vi "config_curve.vi"(10 "簇":T23, 11 "配置":T1 {"串口通信UI"."Format" items=["标准帧", "扩展帧"]; "串口通信UI"."Type" items=["数据帧", "远程帧"]; "串口通信UI"."ID" format="0x%x"; "串口通信UI"."Fliter" items=["接收所有类型"=1, "只接收标准帧"=2, "只接收扩展帧"=3]; "串口通信UI"."kBaudRate" items=["5k bps"=1, "10k bps"=2, "20k bps"=3, "40k bps"=4, "50k bps"=5, "80k bps"=6, "100k bps"=7, "125k bps"=8, "200k bps"=9, "250k bps"=10, "400k bps"=11, "500k bps"=12, "666k bps"=13, "800k bps"=14, "1000k bps"=15, "33.33k bps"=16, "66.66k bps"=17, "83.33k bps"=18]; "串口通信UI"."Mode" items=["正常工作", "仅侦听模式", "自测模式（环回）"]; "串口通信UI"."InitFlag" items=["使用界面设置参数"=1]; "串口通信UI"."AccMask" format="%08x"; "串口通信UI"."AccCode" format="%08x"; "串口通信UI"."Channel" items=["通道1", "通道2"]; "串口通信UI"."DevType" items=["USB-CAN"=3, "USB-CAN2"=4]; "安全报警UI"."操作 8" items=["产生报警信息（不发声），等待手动操作", "产生报警信息（发声），等待手动操作", "产生报警信息（不发声），自动刹车", "产生报警信息（发声），自动刹车", "产生报警信息（不发声），立即自动断电，开启泄放电阻", "产生报警信息（发声），立即自动断电，开启泄放电阻"]; "安全报警UI"."操作 7" items=["产生报警信息（不发声），等待手动操作", "产生报警信息（发声），等待手动操作", "产生报警信息（不发声），自动刹车", "产生报警信息（发声），自动刹车", "产生报警信息（不发声），立即自动断电，开启泄放电阻", "产生报警信息（发声），立即自动断电，开启泄放电阻"]; "安全报警UI"."操作 6" items=["产生报警信息（不发声），等待手动操作", "产生报警信息（发声），等待手动操作", "产生报警信息（不发声），自动刹车", "产生报警信息（发声），自动刹车", "产生报警信息（不发声），立即自动断电，开启泄放电阻", "产生报警信息（发声），立即自动断电，开启泄放电阻"]; "安全报警UI"."操作 5" items=["产生报警信息（不发声），等待手动操作", "产生报警信息（发声），等待手动操作", "产生报警信息（不发声），自动刹车", "产生报警信息（发声），自动刹车", "产生报警信息（不发声），立即自动断电，开启泄放电阻", "产生报警信息（发声），立即自动断电，开启泄放电阻"]; "安全报警UI"."操作 4" items=["产生报警信息（不发声），等待手动操作", "产生报警信息（发声），等待手动操作", "产生报警信息（不发声），自动刹车", "产生报警信息（发声），自动刹车", "产生报警信息（不发声），立即自动断电，开启泄放电阻", "产生报警信息（发声），立即自动断电，开启泄放电阻"]; "安全报警UI"."操作 3" items=["产生报警信息（不发声），等待手动操作", "产生报警信息（发声），等待手动操作", "产生报警信息（不发声），自动刹车", "产生报警信息（发声），自动刹车", "产生报警信息（不发声），立即自动断电，开启泄放电阻", "产生报警信息（发声），立即自动断电，开启泄放电阻"]; "安全报警UI"."操作 2" items=["产生报警信息（不发声），等待手动操作", "产生报警信息（发声），等待手动操作", "产生报警信息（不发声），自动刹车", "产生报警信息（发声），自动刹车", "产生报警信息（不发声），立即自动断电，开启泄放电阻", "产生报警信息（发声），立即自动断电，开启泄放电阻"]; "安全报警UI"."操作" items=["产生报警信息（不发声），等待手动操作", "产生报警信息（发声），等待手动操作", "产生报警信息（不发声），自动刹车", "产生报警信息（发声），自动刹车", "产生报警信息（不发声），立即自动断电，开启泄放电阻", "产生报警信息（发声），立即自动断电，开启泄放电阻"]}) -> (3 "配置输出":T1 {"串口通信UI"."Format" items=["标准帧", "扩展帧"]; "串口通信UI"."Type" items=["数据帧", "远程帧"]; "串口通信UI"."ID" format="0x%x"; "串口通信UI"."Fliter" items=["接收所有类型"=1, "只接收标准帧"=2, "只接收扩展帧"=3]; "串口通信UI"."kBaudRate" items=["5k bps"=1, "10k bps"=2, "20k bps"=3, "40k bps"=4, "50k bps"=5, "80k bps"=6, "100k bps"=7, "125k bps"=8, "200k bps"=9, "250k bps"=10, "400k bps"=11, "500k bps"=12, "666k bps"=13, "800k bps"=14, "1000k bps"=15, "33.33k bps"=16, "66.66k bps"=17, "83.33k bps"=18]; "串口通信UI"."Mode" items=["正常工作", "仅侦听模式", "自测模式（环回）"]; "串口通信UI"."InitFlag" items=["使用界面设置参数"=1]; "串口通信UI"."AccMask" format="%08x"; "串口通信UI"."AccCode" format="%08x"; "串口通信UI"."Channel" items=["通道1", "通道2"]; "串口通信UI"."DevType" items=["USB-CAN"=3, "USB-CAN2"=4]; "安全报警UI"."操作 8" items=["产生报警信息（不发声），等待手动操作", "产生报警信息（发声），等待手动操作", "产生报警信息（不发声），自动刹车", "产生报警信息（发声），自动刹车", "产生报警信息（不发声），立即自动断电，开启泄放电阻", "产生报警信息（发声），立即自动断电，开启泄放电阻"]; "安全报警UI"."操作 7" items=["产生报警信息（不发声），等待手动操作", "产生报警信息（发声），等待手动操作", "产生报警信息（不发声），自动刹车", "产生报警信息（发声），自动刹车", "产生报警信息（不发声），立即自动断电，开启泄放电阻", "产生报警信息（发声），立即自动断电，开启泄放电阻"]; "安全报警UI"."操作 6" items=["产生报警信息（不发声），等待手动操作", "产生报警信息（发声），等待手动操作", "产生报警信息（不发声），自动刹车", "产生报警信息（发声），自动刹车", "产生报警信息（不发声），立即自动断电，开启泄放电阻", "产生报警信息（发声），立即自动断电，开启泄放电阻"]; "安全报警UI"."操作 5" items=["产生报警信息（不发声），等待手动操作", "产生报警信息（发声），等待手动操作", "产生报警信息（不发声），自动刹车", "产生报警信息（发声），自动刹车", "产生报警信息（不发声），立即自动断电，开启泄放电阻", "产生报警信息（发声），立即自动断电，开启泄放电阻"]; "安全报警UI"."操作 4" items=["产生报警信息（不发声），等待手动操作", "产生报警信息（发声），等待手动操作", "产生报警信息（不发声），自动刹车", "产生报警信息（发声），自动刹车", "产生报警信息（不发声），立即自动断电，开启泄放电阻", "产生报警信息（发声），立即自动断电，开启泄放电阻"]; "安全报警UI"."操作 3" items=["产生报警信息（不发声），等待手动操作", "产生报警信息（发声），等待手动操作", "产生报警信息（不发声），自动刹车", "产生报警信息（发声），自动刹车", "产生报警信息（不发声），立即自动断电，开启泄放电阻", "产生报警信息（发声），立即自动断电，开启泄放电阻"]; "安全报警UI"."操作 2" items=["产生报警信息（不发声），等待手动操作", "产生报警信息（发声），等待手动操作", "产生报警信息（不发声），自动刹车", "产生报警信息（发声），自动刹车", "产生报警信息（不发声），立即自动断电，开启泄放电阻", "产生报警信息（发声），立即自动断电，开启泄放电阻"]; "安全报警UI"."操作" items=["产生报警信息（不发声），等待手动操作", "产生报警信息（发声），等待手动操作", "产生报警信息（不发声），自动刹车", "产生报警信息（发声），自动刹车", "产生报警信息（不发声），立即自动断电，开启泄放电阻", "产生报警信息（发声），立即自动断电，开启泄放电阻"]})   [LabVIEW 2018, in "UI.lvlib"]
uses:
  UI.lvlib
  Logging/Logging Configuration.ctl
  Logging/Logging.lvlib
  Acquisition/Signal Type.ctl
  Acquisition/Acquisition.lvlib
  Acquisition/Hardware Configuration.ctl
  Settings/Settings.ctl
  Settings/Settings.lvlib
panel:
  # "参数配置文件"
  # "输入数据文件"
  # "加载电机"
  # "负载电机"
  # "注：每次运行实验时销毁现有所有图像"
  # "参数配置文件"
  # "输入数据文件"
  # "加载电机"
  # "负载电机"
  # "注：每次运行实验时销毁现有所有图像"
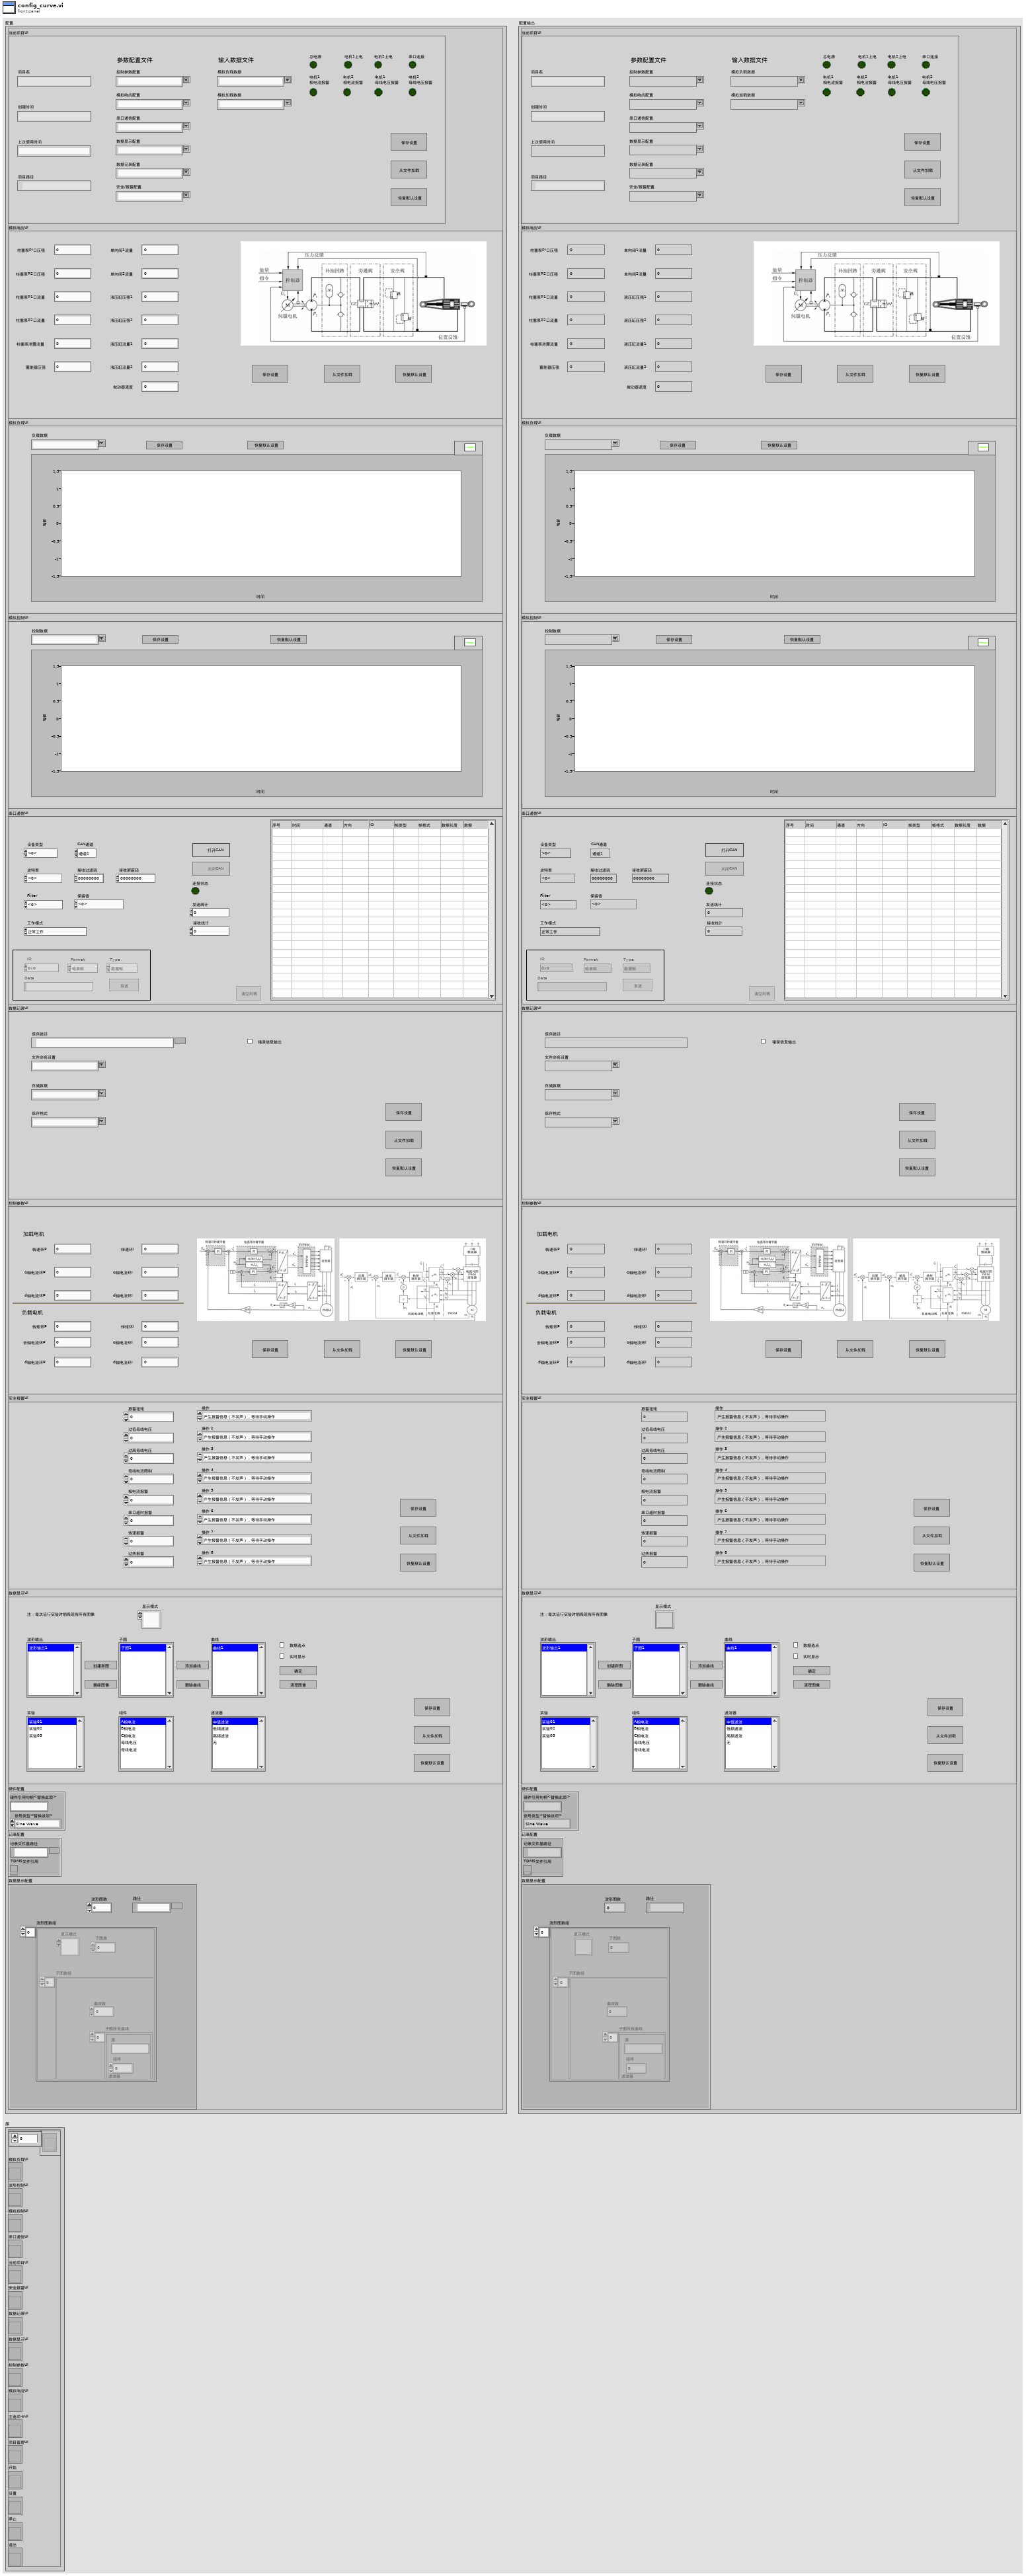
[diagram p1: front panel]
types:
  T1 = typedef "Settings.lvlib/Settings.ctl" = cluster{"当前项目UI":T2, "模拟响应UI":T3, "模拟负载UI":T4, "模拟控制UI":T5, "串口通信UI":T6, "数据记录UI":T12, "控制参数UI":T13, "安全报警UI":T14, "数据显示UI":T15, "硬件配置":T16, "记录配置":T18, "数据显示配置":T19}
  T2 = typedef "控件 5.ctl" = cluster{"控制参数配置":string, "模拟响应配置":string, "串口通信配置":string, "数据显示配置":string, "数据记录配置":string, "安全/报警配置":string, "模拟负载数据":string, "模拟加载数据":string, "总电源":bool, "电机1上电":bool, "电机2上电":bool, "串口连接":bool, "电机1\n相电流报警":bool, "电机2\n相电流报警":bool, "电机1\n母线电压报警":bool, "电机2\n母线电压报警":bool, "保存设置":bool, "从文件加载":bool, "恢复默认设置":bool, "路径":path, "项目路径":path, "项目名":string, "创建时间":string, "上次使用时间":string}
  T3 = typedef "模拟响应UI.ctl" = cluster{"柱塞泵P!口压强":dbl, "柱塞泵P2口压强":dbl, "柱塞泵P1口流量":dbl, "柱塞泵P2口流量":dbl, "柱塞泵泄露流量":dbl, "蓄能器压强":dbl, "单向阀1流量":dbl, "单向阀2流量":dbl, "液压缸压强1":dbl, "液压缸压强2":dbl, "液压缸流量1":dbl, "液压缸流量2":dbl, "做动器速度":dbl, "保存设置":bool, "从文件加载":bool, "恢复默认设置":bool, "路径":path}
  T4 = typedef "控件 9.ctl" = cluster{"负载数据":string, "负载数据 2":waveform(dbl)[], "保存设置":bool, "恢复默认设置":bool}
  T5 = typedef "控件 7.ctl" = cluster{"控制数据":string, "负载数据 2":waveform(dbl)[], "保存设置":bool, "恢复默认设置":bool}
  T6 = typedef "控件 6.ctl" = cluster{"DevType":T7, "Channel":T8, "AccCode":u32, "AccMask":u32, "InitFlag":T9, "Mode":T10, "kBaudRate":u8, "Fliter":T11, "Open":bool, "Close":bool, "连接状态":bool, "SendCnt":u32, "RecvCnt":u32, "Send":bool, "ID":u32, "Data":string, "Type":u8, "Format":u8, "Clear":bool, "list":i32, "路径":path}
  T7 = typedef "ControlCAN.lvlib/DevType.ctl" = u32
  T8 = typedef "ControlCAN.lvlib/CAN Channel.ctl" = u32
  T9 = typedef "ControlCAN.lvlib/InitFlag.ctl" = u32
  T10 = typedef "ControlCAN.lvlib/Mode.ctl" = u8
  T11 = typedef "ControlCAN.lvlib/Fliter.ctl" = u8
  T12 = typedef "控件 3.ctl" = cluster{"保存路径":path, "文件命名设置":string, "存储数据":string, "保存格式":string, "复选框":bool, "保存设置":bool, "从文件加载":bool, "恢复默认设置":bool, "路径":path}
  T13 = typedef "控件 1.ctl" = cluster{"d轴电流环P":dbl, "转速环P":dbl, "q轴电流环P":dbl, "d轴电流环P":dbl, "转矩环P":dbl, "去轴电流环P":dbl, "转速环I":dbl, "q轴电流环I":dbl, "d轴电流环I":dbl, "转矩环I":dbl, "q轴电流环I":dbl, "d轴电流环I":dbl, "保存设置":bool, "从文件加载":bool, "恢复默认设置":bool, "路径":path}
  T14 = typedef "控件 4.ctl" = cluster{"报警扭矩":dbl, "过低母线电压":dbl, "过高母线电压":dbl, "母线电流限制":dbl, "相电流报警":dbl, "串口超时报警":dbl, "转速报警":dbl, "过热报警":dbl, "操作":u16, "操作 2":u16, "操作 3":u16, "操作 4":u16, "操作 5":u16, "操作 6":u16, "操作 7":u16, "操作 8":u16, "保存设置":bool, "从文件加载":bool, "恢复默认设置":bool, "路径":path}
  T15 = typedef "控件 2.ctl" = cluster{"保存设置":bool, "从文件加载":bool, "恢复默认设置":bool, "实验":i32, "波形输出":i32, "组件":i32, "曲线":i32, "滤波器":i32, "删除曲线":bool, "清理图像":bool, "添加曲线":bool, "数据选点":bool, "确定按钮":bool, "实时显示":bool, "子图":i32, "显示模式":u16, "路径":path, "删除图像":bool, "创建新图":bool}
  T16 = typedef "Acquisition.lvlib/Hardware Configuration.ctl" = cluster{"硬件引用句柄<替换此项>":string, "信号类型<替换该项>":T17}
  T17 = typedef "Acquisition.lvlib/Signal Type.ctl" = enum16{"Sine Wave", "Square with Noise"}
  T18 = typedef "Logging.lvlib/Logging Configuration.ctl" = cluster{"记录文件基路径":path, "TDMS文件引用":refnum<k34>}
  T19 = typedef "波形图簇.ctl" = cluster{"波形图数":u32, "波形图数组":T20[], "路径":path}
  T20 = typedef "波形图.ctl" = cluster{"显示模式":u16, "子图数":u32, "子图数组":T21[]}
  T21 = typedef "子图.ctl" = cluster{"子图所有曲线":T22[], "曲线数":u32}
  T22 = typedef "曲线簇.ctl" = cluster{"源":string, "组件":u32, "滤波器":string}
  T23 = typedef "引用簇.ctl" = cluster{"数组":refnum<vi>[], "模拟负载UI":refnum<vi>, "波形控制UI":refnum<vi>, "模拟控制UI":refnum<vi>, "串口通信UI":refnum<vi>, "当前项目UI":refnum<vi>, "安全报警UI":refnum<vi>, "数据记录UI":refnum<vi>, "数据显示UI":refnum<vi>, "控制参数UI":refnum<vi>, "模拟响应UI":refnum<vi>, "主选项卡UI":refnum<vi>, "项目管理UI":refnum<vi>, "开始":refnum<vi>, "设置":refnum<vi>, "停止":refnum<vi>, "退出":refnum<vi>}
  T24 = typedef "组件常量.ctl" = string[]
  T25 = typedef "滤波器常量.ctl" = string[]
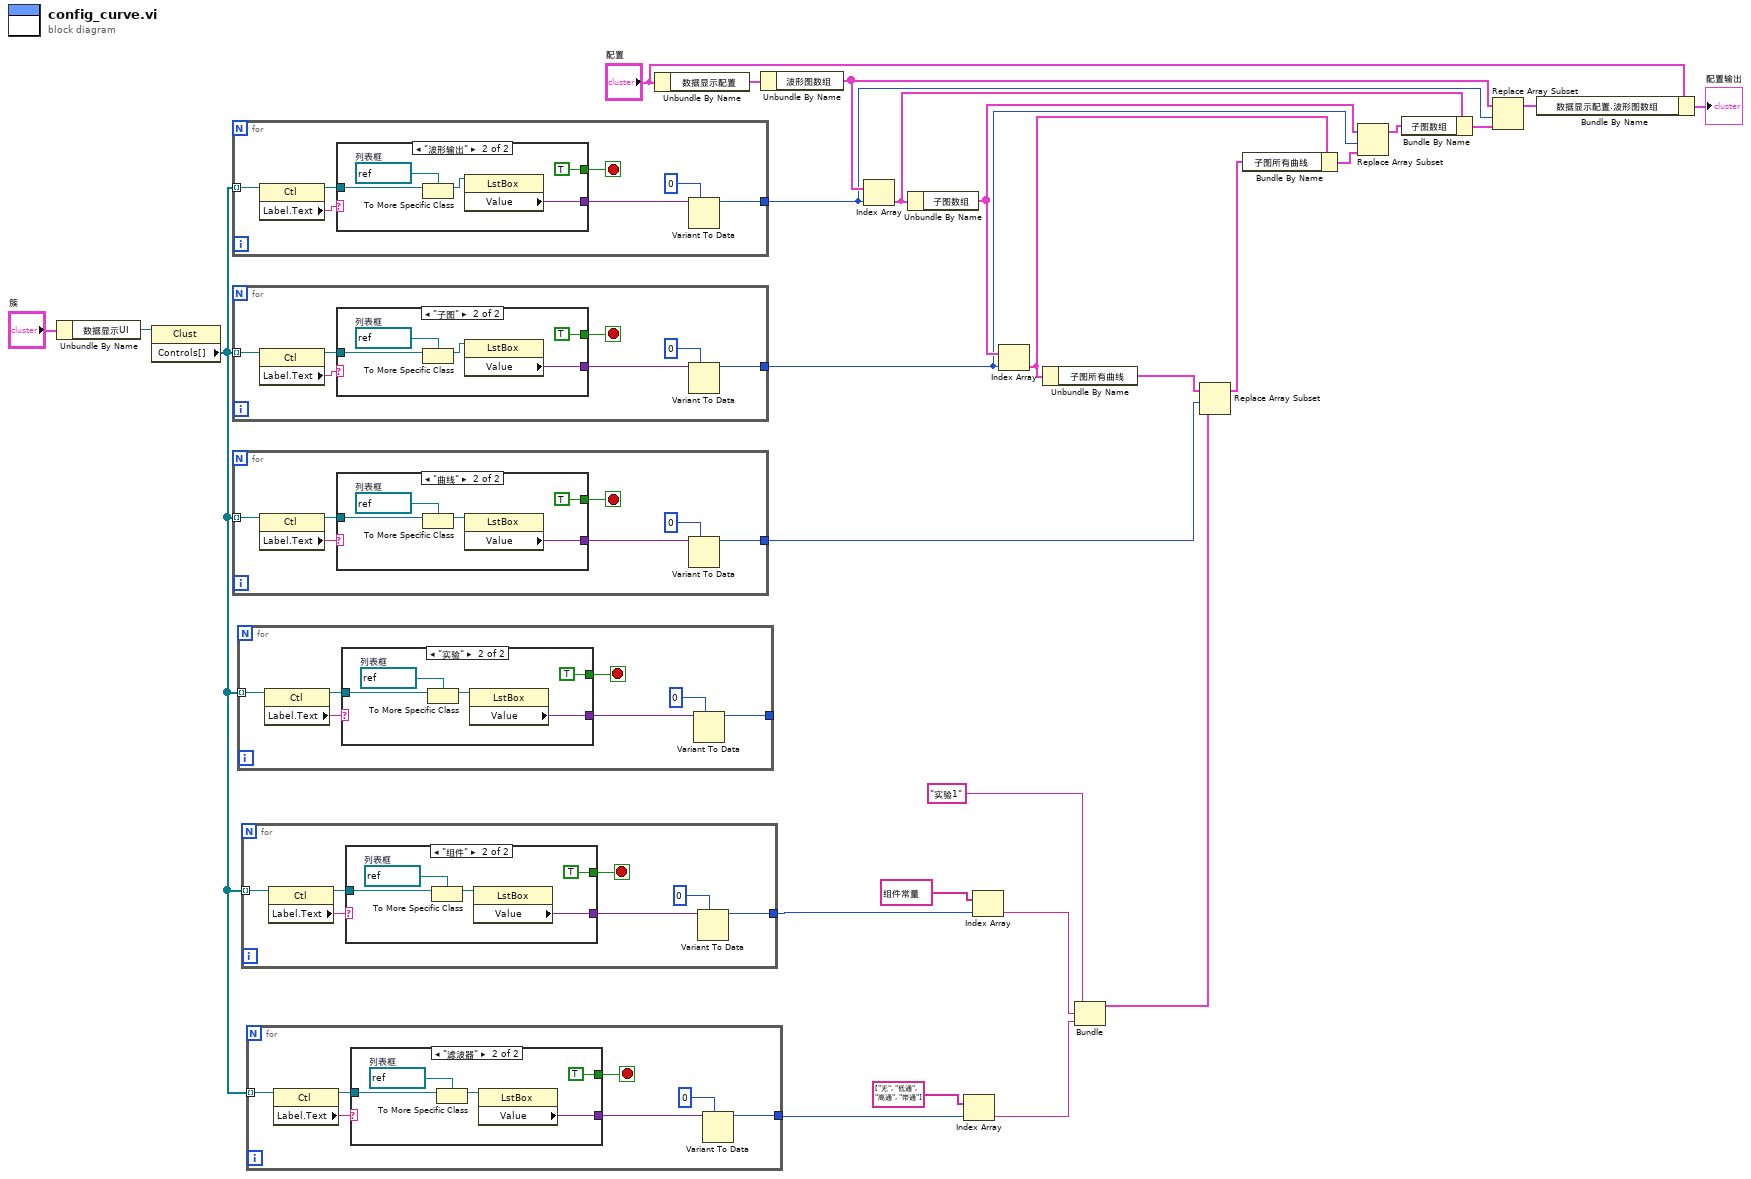
[diagram p0: block diagram]
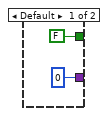
[diagram p2: hidden frame]
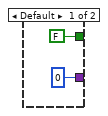
[diagram p3: hidden frame]
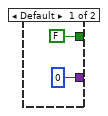
[diagram p4: hidden frame]
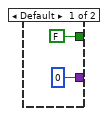
[diagram p5: hidden frame]
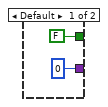
[diagram p6: hidden frame]
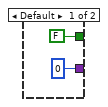
[diagram p7: hidden frame]
diagram:
  n1 = Unbundle By Name("簇") -> ("数据显示UI"=w26:refnum<vi>)
  n2 = property class="Clust"(reference=w26) -> ("Controls[]"=w12:refnum<vi>[])  [unwired: 1 in, 2 out]
  n3 = for {
    tunnel: [w31] -> w20
    tunnel: w12 -> [w28] mode=indexing
    stop <- w29 stop-if-true
    n4 = property class="Ctl"(reference=w28) -> (reference out=w33:refnum<vi>, "Label.Text"=w34:string)  [unwired: 1 in, 1 out]
    n5 = case shown="\"波形输出\"" w34 {
      tunnel: w33 -> [_ w41]
      tunnel: [0 w37] -> w32
      tunnel: [FALSE TRUE] -> w29
      frame Default {
      }
      frame "波形输出" {
        w40 = refnum<vi> refnum  # 列表框
        n6 = To More Specific Class(target class=w40, reference=w41) -> (specific class reference=w39:refnum<vi>)  [unwired: 1 in, 1 out]
        n7 = property class="LstBox"(reference=w39) -> ("Value"=w37:variant)  [unwired: 1 in, 2 out]
      }
    }
    n8 = Variant To Data(type=0, Variant=w32) -> (data=w31:i32)  [unwired: 1 in, 1 out]
  }
  n9 = for {
    tunnel: [w45] -> w24
    tunnel: w12 -> [w42] mode=indexing
    stop <- w43 stop-if-true
    n10 = property class="Ctl"(reference=w42) -> (reference out=w47:refnum<vi>, "Label.Text"=w48:string)  [unwired: 1 in, 1 out]
    n11 = case shown="\"子图\"" w48 {
      tunnel: w47 -> [_ w55]
      tunnel: [0 w51] -> w46
      tunnel: [FALSE TRUE] -> w43
      frame Default {
      }
      frame "子图" {
        w54 = refnum<vi> refnum  # 列表框
        n12 = To More Specific Class(target class=w54, reference=w55) -> (specific class reference=w53:refnum<vi>)  [unwired: 1 in, 1 out]
        n13 = property class="LstBox"(reference=w53) -> ("Value"=w51:variant)  [unwired: 1 in, 2 out]
      }
    }
    n14 = Variant To Data(type=0, Variant=w46) -> (data=w45:i32)  [unwired: 1 in, 1 out]
  }
  n15 = for {
    tunnel: [w59] -> w10
    tunnel: w12 -> [w56] mode=indexing
    stop <- w57 stop-if-true
    n16 = property class="Ctl"(reference=w56) -> (reference out=w61:refnum<vi>, "Label.Text"=w62:string)  [unwired: 1 in, 1 out]
    n17 = case shown="\"曲线\"" w62 {
      tunnel: w61 -> [_ w69]
      tunnel: [0 w65] -> w60
      tunnel: [FALSE TRUE] -> w57
      frame Default {
      }
      frame "曲线" {
        w68 = refnum<vi> refnum  # 列表框
        n18 = To More Specific Class(target class=w68, reference=w69) -> (specific class reference=w67:refnum<vi>)  [unwired: 1 in, 1 out]
        n19 = property class="LstBox"(reference=w67) -> ("Value"=w65:variant)  [unwired: 1 in, 2 out]
      }
    }
    n20 = Variant To Data(type=0, Variant=w60) -> (data=w59:i32)  [unwired: 1 in, 1 out]
  }
  n21 = for {
    tunnel: [w73] -> _
    tunnel: w12 -> [w70] mode=indexing
    stop <- w71 stop-if-true
    n22 = property class="Ctl"(reference=w70) -> (reference out=w75:refnum<vi>, "Label.Text"=w76:string)  [unwired: 1 in, 1 out]
    n23 = case shown="\"实验\"" w76 {
      tunnel: w75 -> [_ w83]
      tunnel: [0 w79] -> w74
      tunnel: [FALSE TRUE] -> w71
      frame Default {
      }
      frame "实验" {
        w82 = refnum<vi> refnum  # 列表框
        n24 = To More Specific Class(target class=w82, reference=w83) -> (specific class reference=w81:refnum<vi>)  [unwired: 1 in, 1 out]
        n25 = property class="LstBox"(reference=w81) -> ("Value"=w79:variant)  [unwired: 1 in, 2 out]
      }
    }
    n26 = Variant To Data(type=0, Variant=w74) -> (data=w73:i32)  [unwired: 1 in, 1 out]
  }
  n27 = for {
    tunnel: [w87] -> w6
    tunnel: w12 -> [w84] mode=indexing
    stop <- w85 stop-if-true
    n28 = property class="Ctl"(reference=w84) -> (reference out=w89:refnum<vi>, "Label.Text"=w90:string)  [unwired: 1 in, 1 out]
    n29 = case shown="\"组件\"" w90 {
      tunnel: w89 -> [_ w97]
      tunnel: [0 w93] -> w88
      tunnel: [FALSE TRUE] -> w85
      frame Default {
      }
      frame "组件" {
        w96 = refnum<vi> refnum  # 列表框
        n30 = To More Specific Class(target class=w96, reference=w97) -> (specific class reference=w95:refnum<vi>)  [unwired: 1 in, 1 out]
        n31 = property class="LstBox"(reference=w95) -> ("Value"=w93:variant)  [unwired: 1 in, 2 out]
      }
    }
    n32 = Variant To Data(type=0, Variant=w88) -> (data=w87:i32)  [unwired: 1 in, 1 out]
  }
  n33 = for {
    tunnel: [w101] -> w8
    tunnel: w12 -> [w98] mode=indexing
    stop <- w99 stop-if-true
    n34 = property class="Ctl"(reference=w98) -> (reference out=w103:refnum<vi>, "Label.Text"=w104:string)  [unwired: 1 in, 1 out]
    n35 = case shown="\"滤波器\"" w104 {
      tunnel: w103 -> [_ w111]
      tunnel: [0 w107] -> w102
      tunnel: [FALSE TRUE] -> w99
      frame Default {
      }
      frame "滤波器" {
        w110 = refnum<vi> refnum  # 列表框
        n36 = To More Specific Class(target class=w110, reference=w111) -> (specific class reference=w109:refnum<vi>)  [unwired: 1 in, 1 out]
        n37 = property class="LstBox"(reference=w109) -> ("Value"=w107:variant)  [unwired: 1 in, 2 out]
      }
    }
    n38 = Variant To Data(type=0, Variant=w102) -> (data=w101:i32)  [unwired: 1 in, 1 out]
  }
  n39 = Unbundle By Name("配置") -> ("数据显示配置"=w27:T19)
  n40 = Unbundle By Name(w27) -> ("波形图数组"=w21:T20[])
  n41 = Index Array(array=w21, index=w20) -> (element=w23:T20)
  n42 = Unbundle By Name(w23) -> ("子图数组"=w25:T21[])
  n43 = Index Array(array=T25 ["无", "低通", "高通", "带通"] ("数组"), index=w8) -> (element=w5:string)
  n44 = Index Array(array=T24 ["正弦", "方波", "三角", "锯齿"] ("数组"), index=w6) -> (element=w4:string)
  n45 = Index Array(array=w25, index=w24) -> (element=w17:T21)
  n46 = Unbundle By Name(w17) -> ("子图所有曲线"=w11:T22[])
  n47 = Bundle("实验1", w4, w5) -> (w2:cluster{string, string, string})  [unwired: 1 in]
  n48 = Replace Array Subset(array=w11, new element=w2, index=w10) -> (w1:T22[])
  n49 = Bundle By Name(cluster=w17, "子图所有曲线"=w1) -> (w16:T21)
  n50 = Replace Array Subset(array=w25, new element=w16, index=w24) -> (w22:T21[])
  n51 = Bundle By Name(cluster=w23, "子图数组"=w22) -> (w19:T20)
  n52 = Replace Array Subset(array=w21, new element=w19, index=w20) -> (w18:T20[])
  n53 = Bundle By Name(cluster="配置", "数据显示配置.波形图数组"=w18) -> (→"配置输出":T1)
